vi "IT8900A-E Series Create and Save List File.vi"() -> ()   [LabVIEW 2015]
uses:
  <instrlib>/IT8900/IT8900A-E.lvlib
panel:
  in  "Step Level (1)":dbl[](array[numeric]) min=1.0 max=999.99 step=0.01 format="%.4g"
  in  "Step Width (1)":dbl[](array[numeric]) min=2e-05 max=3600.0 step=1.0 format="%.3g"
  in  "Step Slew Rate (0.1)":dbl[](array[numeric]) min=0.0001 max=65536.0 step=0.0001 format="%.4g"
  in  "List Number (1)":dbl=1.0 min=1.0 max=7.0 format="%#_0f"
  in  "Total Steps (2)":dbl=2.0 min=2.0 max=84.0 step=1.0 format="%.0g"
  in  "List Count (1)":dbl=1.0 min=1.0 max=65536.0 step=1.0 format="%.0g"
  in  "Range (20)":dbl=20.0001 min=0.0001 max=120.0 step=1.0 format="%.2g"
  in  "Serial Configuration":cluster{"Baud Rate":u32}={"Baud Rate"=9600} {"Baud Rate" items=["300"=300, "600"=600, "1200"=1200, "2400"=2400, "4800"=4800, "9600"=9600, "19200"=19200]}
  in  "VISA resource name":refnum<visa-resource-name>
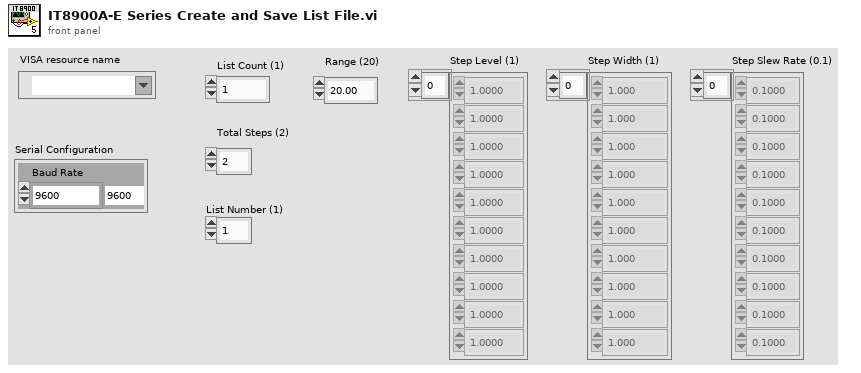
[diagram p1: front panel]
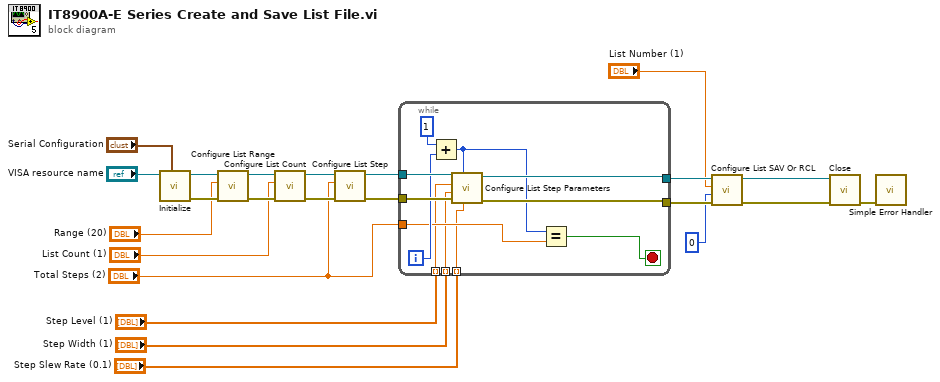
[diagram p0: block diagram]
diagram:
  n1 = call <instrlib>:"Initialize.vi"("Serial Configuration"="Serial Configuration", "VISA resource name"="VISA resource name") -> ("error out"=w20:errorcluster, "VISA resource name out"=w19:refnum<visa-resource-name>)  [unwired: 8 in]
  n2 = call <instrlib>:"Configure List Range.vi"("error in (no error)"=w20, "Range"="Range (20)", "VISA resource name"=w19) -> ("error out"=w18:errorcluster, "VISA resource name out"=w17:refnum<visa-resource-name>)  [unwired: 7 in]
  n3 = call <instrlib>:"Configure List Count.vi"("error in (no error)"=w18, "Count  : 1-65536"="List Count (1)", "VISA resource name"=w17) -> ("error out"=w16:errorcluster, "VISA resource name out"=w15:refnum<visa-resource-name>)  [unwired: 7 in]
  n4 = call <instrlib>:"Configure List Step.vi"("error in (no error)"=w16, "Setp  : 2 - 80"="Total Steps (2)", "VISA resource name"=w15) -> ("error out"=w9:errorcluster, "VISA resource name out"=w10:refnum<visa-resource-name>)  [unwired: 7 in]
  n5 = while {
    tunnel: [w33] -> w12
    tunnel: [w32] -> w11
    tunnel: w10 -> [w35]
    tunnel: w9 -> [w34]
    tunnel: "Total Steps (2)" -> [w28]
    tunnel: "Step Level (1)" -> [w26] mode=indexing
    tunnel: "Step Width (1)" -> [w25] mode=indexing
    tunnel: "Step Slew Rate (0.1)" -> [w24] mode=indexing
    i -> [w31]
    stop <- w27 stop-if-true
    n6 = Add(x=1, y=w31) -> (x+y=w29:i32)
    n7 = call <instrlib>:"Configure List Step Parameters.vi"("Step Slew Rate (1)"=w24, "Step Number (1)"=w29, "error in (no error)"=w34, "Step Width (1)"=w25, "Step Level (1)"=w26, "VISA resource name"=w35) -> ("error out"=w32:errorcluster, "VISA resource name out"=w33:refnum<visa-resource-name>)  [unwired: 4 in]
    n8 = Equal?(x=w29, y=w28) -> (x = y?=w27:bool)
  }
  n9 = call <instrlib>:"Configure List SAV Or RCL.vi"("error in (no error)"=w11, "Save Type ( 0 : Save)"=0, "File Add ( 1 - 5 )"="List Number (1)", "VISA resource name"=w12) -> ("error out"=w7:errorcluster, "VISA resource name out"=w8:refnum<visa-resource-name>)  [unwired: 6 in]
  n10 = call <instrlib>:"Close.vi"("error in (no error)"=w7, "VISA resource name"=w8) -> ("error out"=w23:errorcluster)  [unwired: 9 in]
  n11 = call <vilib>:"Simple Error Handler.vi"("error in (no error)"=w23) -> ()  [unwired: 4 in, 5 out]
